vi "vms_getNextSample_TMA.vi"(8 "error in (no error)":errorcluster, 11 "TMA_Ctl":T1) -> (0 "error out":errorcluster, 2 "function return":i32, 3 "TMA_Ctl out":T1)   [LabVIEW 2016, in "SALLV_vms.lvlib"]
doc: "int vms_shm_getNextSample_TMALV(vms_TMALV *TMA_Ctl );"
uses:
  SALLV_vms.lvlib
  DataTypes/TMA.ctl
  SALLV_vms.so
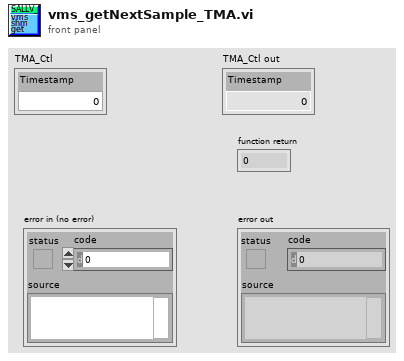
[diagram p1: front panel]
types:
  T1 = typedef "SALLV_vms.lvlib/TMA.ctl" = cluster{"Timestamp":dbl}
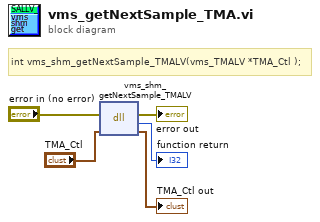
[diagram p0: block diagram]
diagram:
  # "int vms_shm_getNextSample_TMALV(vms_TMALV *TMA_Ctl );"
  n1 = dll-call lib="opt/CODE/SALLV_vms/SALLV_vms.*" fn="vms_shm_getNextSample_TMALV"(error in="error in (no error)", "TMA_Ctl"="TMA_Ctl") -> (error out=→"error out":errorcluster, →"function return":i32, "TMA_Ctl"=→"TMA_Ctl out":T1)  [unwired: 2 in, 1 out]
